vi "check.if.done.vi"(8 "error in (no error)":errorcluster, 11 "comic_crawler in":refnum<class "comic_crawler.lvclass">) -> (0 "error out":errorcluster, 3 "comic_crawler out":refnum<class "comic_crawler.lvclass">)   [LabVIEW 2024, in "comic_crawler.lvclass"]
uses:
  comic_crawler.lvclass
  daemon.states--enum.ctl
  comic_crawler.lvclass/comic_crawler.ctl
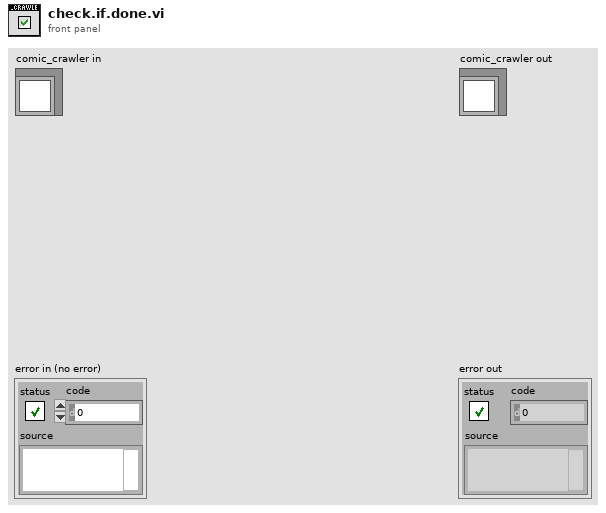
[diagram p1: front panel]
types:
  T1 = typedef "comic_crawler.lvclass/daemon.states--enum.ctl" = enum16{"start search", "idle", "set timer", "running", "stop search", "wait", "set delay", "shut down"}
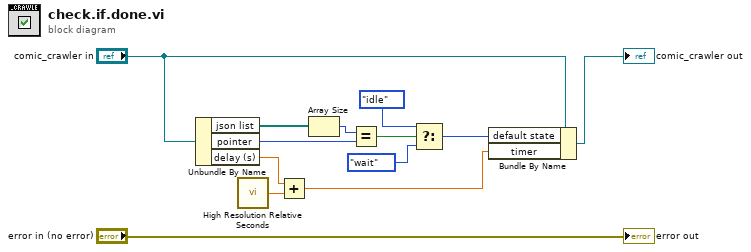
[diagram p0: block diagram]
diagram:
  n1 = Unbundle By Name("comic_crawler in") -> ("json list"=w10:path[], "pointer"=w8:i32, "delay (s)"=w3:dbl)
  n2 = call <vilib>:"High Resolution Relative Seconds.vi"() -> ("relative seconds"=w4:dbl)
  n3 = Add(x=w3, y=w4) -> (x+y=w1:dbl)
  n4 = Array Size(array=w10) -> (size(s)=w9:i32)
  n5 = Equal?(x=w9, y=w8) -> (x = y?=w7:bool)
  n6 = Select(t=daemon.states--enum."idle" ("states"), s=w7, f=daemon.states--enum."wait") -> (s? t:f=w5:T1)
  n7 = Bundle By Name(cluster="comic_crawler in", "default state"=w5, "timer"=w1) -> (→"comic_crawler out":refnum<class "comic_crawler.lvclass">)
  "error out" <- "error in (no error)"
